vi "set Data Store.vi"(8 "error in (no error)":errorcluster, 10 "Data Store":refnum<data-value>, 11 "Actor in":refnum<class "Actor.lvclass">) -> (0 "error out":errorcluster, 3 "Actor out":refnum<class "Actor.lvclass">)   [LabVIEW 2015]
uses:
  Actor.lvclass
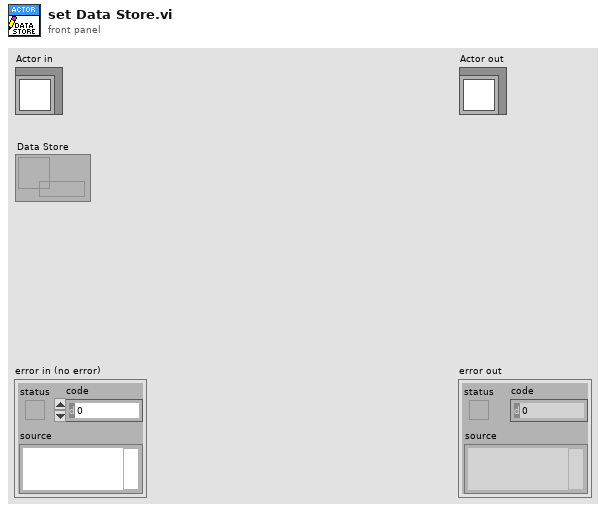
[diagram p1: front panel]
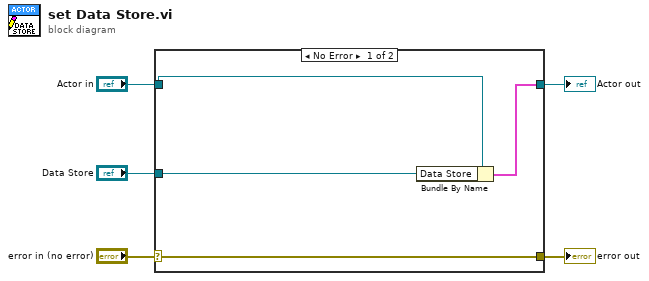
[diagram p0: block diagram]
diagram:
  n1 = case shown="No Error" "error in (no error)" {
    selector: "error in (no error)" -> [w9 w10]
    tunnel: [w9 w10] -> w4
    tunnel: [w7 w11] -> w2
    tunnel: "Actor in" -> [w8 w11]
    tunnel: "Data Store" -> [w6 _]
    frame No Error {
      n2 = Bundle By Name(cluster=w8, "Data Store"=w6) -> (w7:cluster{})
    }
    frame Error {
    }
  }
  "error out" <- w4
  "Actor out" <- w2
